vi "get_stored_setpoint.vi"(8 "error in (no error)":errorcluster, 9 "connection information":path, 10 "output channel":refnum<k21>, 11 "heat_board_control in":refnum<class "heat_board_control.lvclass">) -> (0 "error out":errorcluster, 2 "setpoint":dbl, 3 "heat_board_control out":refnum<class "heat_board_control.lvclass">)   [LabVIEW 2015, in "heat_board_control.lvclass"]
uses:
  heat_board_control.lvclass
  <vilib>/addons/database/Connection.llb/DB Tools Open Connec (Path).vi
  <vilib>/addons/database/_DB Variant To Data/Database Variant To Data.xnode
  <vilib>/addons/database/NI_Database_API.lvlib
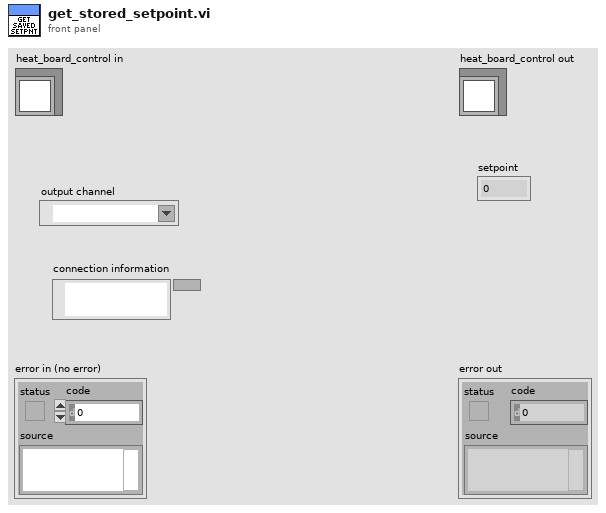
[diagram p1: front panel]
types:
  T1 = typedef "NI_Database_API.lvlib/Conn ObjectReference.ctl" = refnum<k1>
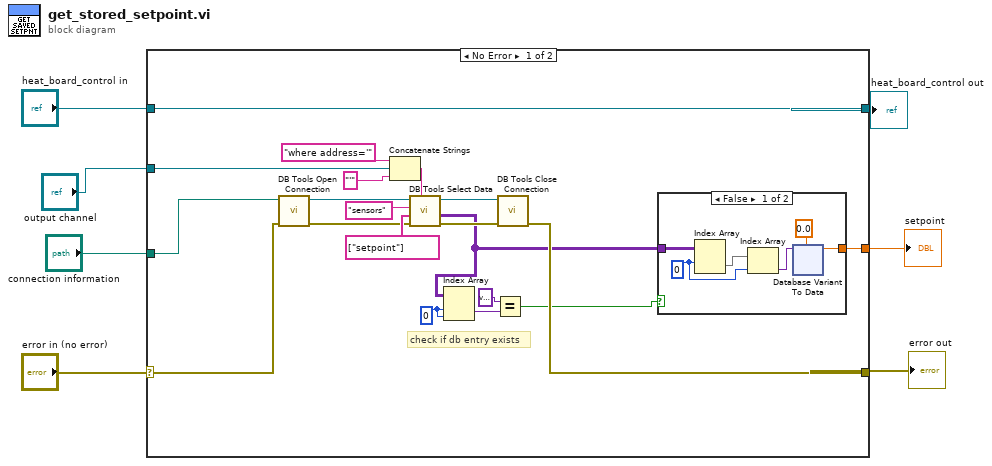
[diagram p0: block diagram]
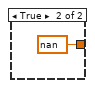
[diagram p2: hidden frame]
diagram:
  n1 = case shown="No Error" "error in (no error)" {
    selector: "error in (no error)" -> [w15 w68]
    tunnel: [w14 w68] -> w6
    tunnel: [w27 w67] -> w4
    tunnel: "heat_board_control in" -> [w27 w67]
    tunnel: "connection information" -> [w23 _]
    tunnel: "output channel" -> [w17 _]
    tunnel: [w13 _] -> w1
    frame No Error {
      w12 = 0
      # "check if db entry exists"
      n2 = call-poly <vilib>:"DB Tools Open Connection.vi"("error in (no error)"=w15, "connection information"=w23) -> ("error out"=w21:errorcluster, "connection reference"=w22:T1)  [unwired: 6 in]
      n3 = Concatenate Strings("where address='" ("condition"), w17, "'") -> (w19:string)
      n4 = call <vilib>:"DB Tools Select Data.vi"("condition"=w19, "error in (no error)"=w21, "columns"=string[] ["setpoint"], "table"="sensors", "connection reference"=w22) -> ("error out"=w16:errorcluster, "data"=w9:variant[][], "connection reference out"=w26:T1)  [unwired: 1 in]
      n5 = Index Array(array=w9, index (row)=w12, index (col)=w12) -> (element=w11:variant)
      n6 = Equal?(x=variant ("y"), y=w11) -> (x = y?=w8:bool)
      n7 = call <vilib>:"DB Tools Close Connection.vi"("error in (no error)"=w16, "connection reference"=w26) -> ("error out"=w14:errorcluster)  [unwired: 5 in]
      n8 = case shown="False" w8 {
        tunnel: w9 -> [w31 _]
        tunnel: [w30 nan ("data")] -> w13
        frame False {
          w32 = 0
          n9 = Index Array(array=w31, index (row)=w32) -> (element=w33:variant[])  [unwired: 1 in]
          n10 = Index Array(array=w33, index=w32) -> (element=w29:variant)
          n11 = xnode "Database Variant To Data"("database variant"=w29, "type"=0.0) -> ("data"=w30:dbl)  [unwired: 1 in, 1 out]
        }
        frame True {
        }
      }
    }
    frame Error {
    }
  }
  "error out" <- w6
  "heat_board_control out" <- w4
  "setpoint" <- w1
